vi "Check If Software On Target.vi"(10 "installed software":T1[](array[typedef]) {"component type" items=["standard", "hidden", "system", "unknown", "startup", "image"]}, 11 "software to check":T1[](array[typedef]) {"component type" items=["standard", "hidden", "system", "unknown", "startup", "image"]}) -> (2 "missing software":T1[](array[typedef]) {"component type" items=["standard", "hidden", "system", "unknown", "startup", "image"]}, 3 "software installed":bool)   [LabVIEW 2013]
uses:
  <vilib>/nisyscfg/Software 1.2.ctl
  <vilib>/nisyscfg/Component Type.ctl
  <vilib>/nisyscfg/nisyscfg.lvlib
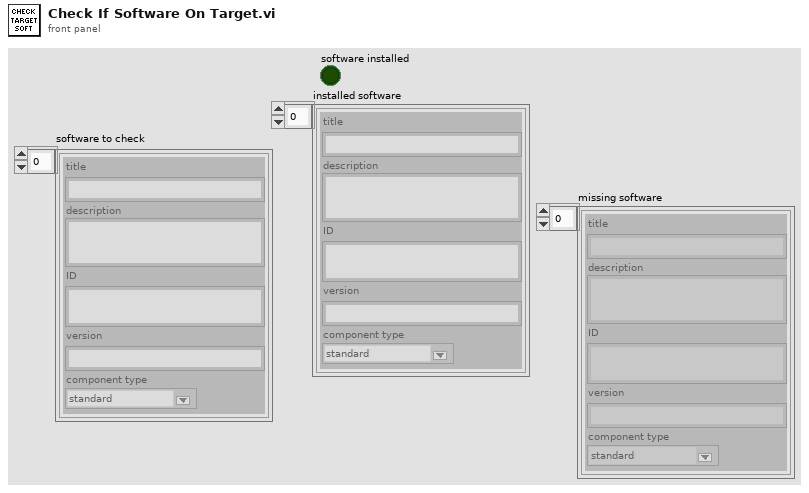
[diagram p1: front panel]
types:
  T1 = typedef "nisyscfg.lvlib/Software 1.2.ctl" = cluster{"title":string, "description":string, "ID":string, "version":string, "component type":T2}
  T2 = typedef "nisyscfg.lvlib/Component Type.ctl" = u32
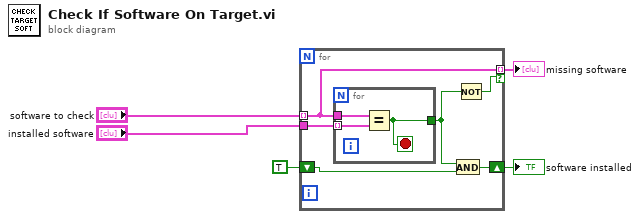
[diagram p0: block diagram]
diagram:
  n1 = for {
    tunnel: "installed software" -> [w11]
    tunnel: "software to check" -> [w10] mode=indexing
    tunnel: [w10] -> w4 mode=indexing if=w9
    shift-right: [w8] -> w2
    shift-left: TRUE -> [w6]
    n2 = for {
      tunnel: w11 -> [w14] mode=indexing
      tunnel: w10 -> [w13]
      tunnel: [w12] -> w7
      stop <- w12 stop-if-true
      n3 = Equal?(x=w13, y=w14) -> (x = y?=w12:bool)
    }
    n4 = And(x=w7, y=w6) -> (x .and. y?=w8:bool)
    n5 = Not(x=w7) -> (.not. x?=w9:bool)
  }
  "missing software" <- w4
  "software installed" <- w2
